vi "Populate Tree View.vi"(7 "Tree":refnum<vi>, 8 "error in (no error)":errorcluster, 11 "Element":refnum<class "Config Element.lvclass">) -> (0 "error out":errorcluster)   [LabVIEW 2020, in "CDM-Config.lvlib"]
doc: "Helper VI to populate a tree control with the specified config tree, starting with the specified [sub]tree root <b>Element</b>. This VI Defers Panel Updates on the owning VI of the <b>Tree</b> while updating the tree to increase performance."
uses:
  CDM-Config.lvlib
  Config Element/Config Element.lvclass
  Config Element/Config Element.lvclass/Config Element.ctl
  0270a6bc-9e24-4c23-b336-e1204a0f26d3.vi
  <vilib>/AdvancedString/1D String Array to Delimited String.vi
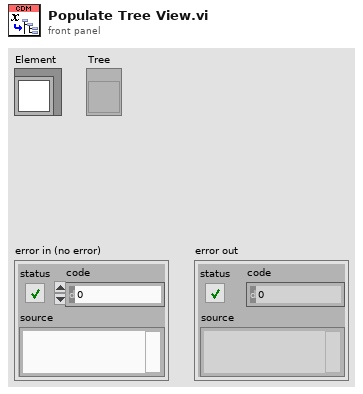
[diagram p1: front panel]
types:
  T1 = typedef "CDM-Config.lvlib/Meta Data.ctl" = cluster{"Name":string, "Value":string}
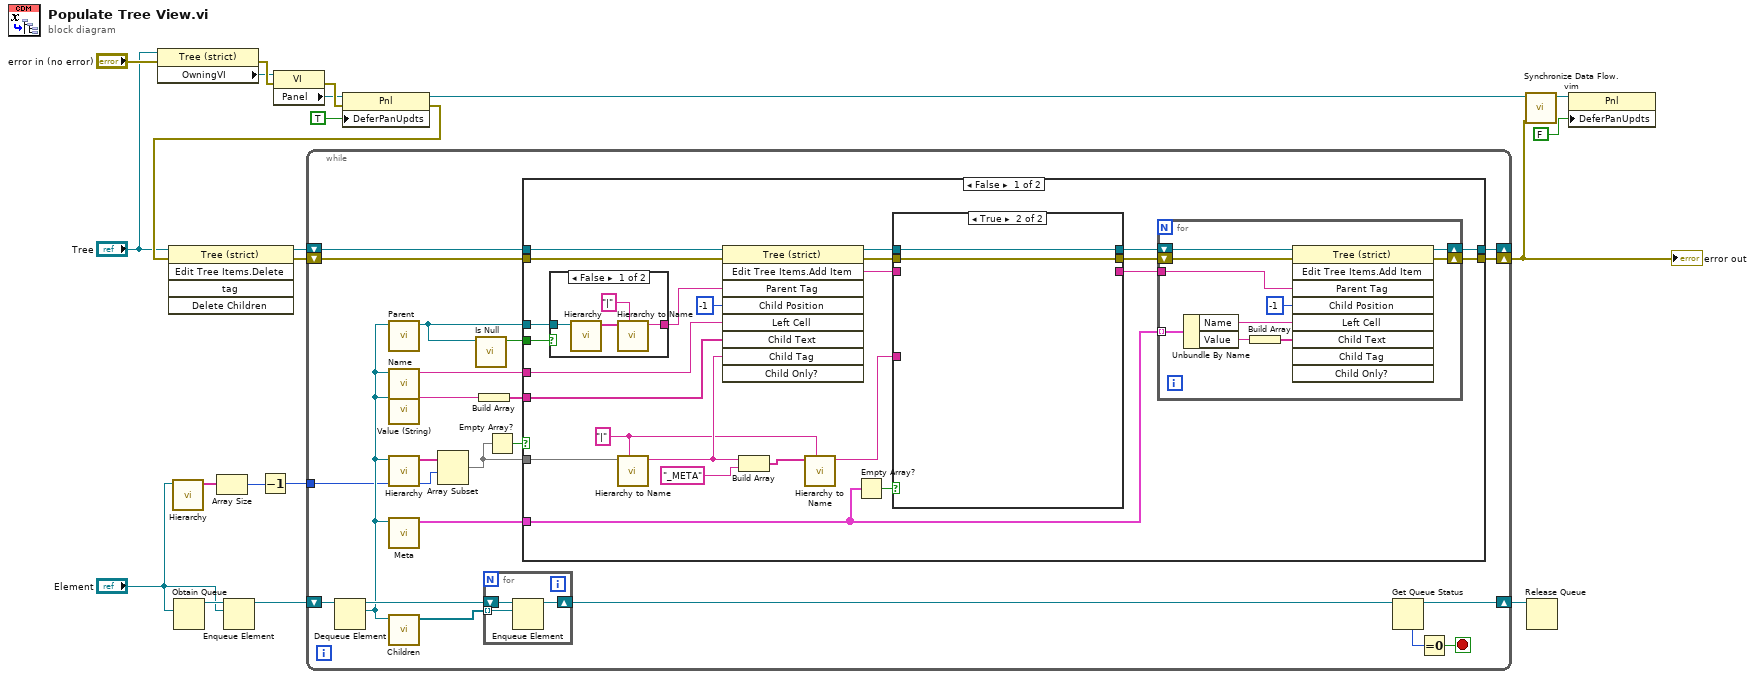
[diagram p0: block diagram]
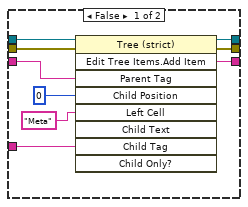
[diagram p3: hidden frame]
diagram:
  n1 = property class="Tree (strict)"(reference="Tree", error in="error in (no error)") -> (error out=w20:errorcluster, "OwningVI"=w12:refnum<vi>)  [unwired: 1 out]
  n2 = call "Hierarchy.vi"("Config Element in"="Element") -> ("Hierarchy"=w3:string[])  [unwired: 9 in, 1 out]
  n3 = Obtain Queue(element data type="Element") -> (queue out=w17:refnum<queue>)  [unwired: 4 in, 2 out]
  n4 = Array Size(array=w3) -> (size(s)=w2:i32)
  n5 = Enqueue Element(queue=w17, element="Element") -> (queue out=w16:refnum<queue>)  [unwired: 2 in, 2 out]
  n6 = Decrement(x=w2) -> (x-1=w1:i32)
  n7 = property class="VI"(reference=w12, error in=w20) -> (error out=w19:errorcluster, "Panel"=w11:refnum<vi>)  [unwired: 1 out]
  n8 = property class="Pnl"(reference=w11, error in=w19, "DeferPanUpdts"=TRUE ("Defer Panel Updates")) -> (reference out=w9:refnum<vi>, error out=w18:errorcluster)
  n9 = invoke class="Tree (strict)" method="Edit Tree Items.Delete"(reference="Tree", error in=w18) -> (reference out=w15:refnum<vi>, error out=w14:errorcluster)  [unwired: 3 in, 3 out]
  n10 = while {
    shift-right: [w42] -> w5
    shift-left: w16 -> [w43]
    shift-right: [w31] -> _
    shift-left: w15 -> [w36]
    shift-right: [w30] -> w7
    shift-left: w14 -> [w35]
    tunnel: w1 -> [w22]
    stop <- w39 stop-if-true
    n11 = Dequeue Element(queue=w43) -> (queue out=w41:refnum<queue>, element=w29:refnum<class "Config Element.lvclass">)  [unwired: 2 in, 2 out]
    n12 = call "Parent.vi"("Config Element in"=w29) -> ("Parent"=w33:refnum<class "Config Element.lvclass">)  [unwired: 9 in, 1 out]
    n13 = call "Name.vi"("Config Element in"=w29) -> ("Name"=w32:string)  [unwired: 9 in, 1 out]
    n14 = call "Value (String).vi"("Config Element in"=w29) -> ("String Value"=w28:string)  [unwired: 9 in, 1 out]
    n15 = call "Hierarchy.vi"("Config Element in"=w29) -> ("Hierarchy"=w24:string[])  [unwired: 9 in, 1 out]
    n16 = call "Meta.vi"("Config Element in"=w29) -> ("Meta Data"=w26:T1[])  [unwired: 9 in, 1 out]
    n17 = call "Children.vi"("Config Element in"=w29) -> ("Elements"=w37:refnum<class "Config Element.lvclass">[])  [unwired: 9 in, 1 out]
    n18 = Array Subset(array=w24, index=w22) -> (w23:string[])  [unwired: 1 in]
    n19 = call "Is Null.vi"("Config Element in"=w33) -> ("Null"=w34:bool)  [unwired: 10 in]
    n20 = Build Array(w28) -> (w27:string[])
    n21 = for {
      shift-right: [w96] -> w38
      shift-left: w41 -> [w97]
      tunnel: w37 -> [w95] mode=indexing
      n22 = Enqueue Element(queue=w97, element=w95) -> (queue out=w96:refnum<queue>)  [unwired: 2 in, 2 out]
    }
    n23 = Empty Array?(array=w23) -> (empty?=w25:bool)
    n24 = case shown="False" w25 {
      tunnel: w36 -> [w67 w94]
      tunnel: w35 -> [w66 w93]
      tunnel: w34 -> [w65 _]
      tunnel: w33 -> [w64 _]
      tunnel: w32 -> [w62 _]
      tunnel: [w61 w94] -> w31
      tunnel: [w60 w93] -> w30
      tunnel: w27 -> [w47 _]
      tunnel: w26 -> [w45 _]
      tunnel: w23 -> [w44 _]
      frame False {
        w52 = "|" ("Delimiter")
        n25 = case shown="False" w65 {
          tunnel: w64 -> [w69 _]
          tunnel: [w68 _] -> w63
          frame False {
            n26 = call "Hierarchy.vi"("Config Element in"=w69) -> ("Hierarchy"=w70:string[])  [unwired: 9 in, 1 out]
            n27 = call "Hierarchy to Name.vi"("Delimiter"="|", "Hierarchy"=w70) -> ("Full Name"=w68:string)  [unwired: 9 in]
          }
          frame True {
          }
        }
        n28 = call "Hierarchy to Name.vi"("Delimiter"=w52, "Hierarchy"=w44) -> ("Full Name"=w59:string)  [unwired: 9 in]
        n29 = invoke class="Tree (strict)" method="Edit Tree Items.Add Item"(reference=w67, error in=w66, "Parent Tag"=w63, "Child Position"=-1, "Left Cell"=w62, "Child Text"=w47, "Child Tag"=w59) -> (reference out=w56:refnum<vi>, error out=w55:errorcluster, "Edit Tree Items:Add Item"=w54:string)  [unwired: 2 in, 6 out]
        n30 = Build Array(w59, "_META" ("element")) -> (w53:string[])
        n31 = call "Hierarchy to Name.vi"("Delimiter"=w52, "Hierarchy"=w53) -> ("Full Name"=w51:string)  [unwired: 9 in]
        n32 = Empty Array?(array=w45) -> (empty?=w57:bool)
        n33 = case shown="True" w57 {
          tunnel: w56 -> [w80 w82]
          tunnel: w55 -> [w79 w81]
          tunnel: w54 -> [w78 _]
          tunnel: w51 -> [w73 _]
          tunnel: [w77 _] -> w50
          tunnel: [w76 w82] -> w49
          tunnel: [w75 w81] -> w48
          frame False {
            n34 = invoke class="Tree (strict)" method="Edit Tree Items.Add Item"(reference=w80, error in=w79, "Parent Tag"=w78, "Child Position"=0, "Left Cell"="Meta" ("Left Cell String"), "Child Tag"=w73) -> (reference out=w76:refnum<vi>, error out=w75:errorcluster, "Edit Tree Items:Add Item"=w77:string)  [unwired: 3 in, 6 out]
          }
          frame True {
          }
        }
        n35 = for {
          shift-right: [w87] -> w61
          shift-left: w49 -> [w91]
          shift-right: [w86] -> w60
          shift-left: w48 -> [w90]
          tunnel: w45 -> [w92] mode=indexing
          tunnel: w50 -> [w89]
          n36 = Unbundle By Name(w92) -> ("Name"=w88:string, "Value"=w85:string)
          n37 = Build Array(w85) -> (w84:string[])
          n38 = invoke class="Tree (strict)" method="Edit Tree Items.Add Item"(reference=w91, error in=w90, "Parent Tag"=w89, "Child Position"=-1, "Left Cell"=w88, "Child Text"=w84) -> (reference out=w87:refnum<vi>, error out=w86:errorcluster)  [unwired: 3 in, 7 out]
        }
      }
      frame True {
      }
    }
    n39 = Get Queue Status(queue=w38) -> (queue out=w42:refnum<queue>, # elements in queue=w40:i32)  [unwired: 2 in, 6 out]
    n40 = Equal To 0?(x=w40) -> (x = 0?=w39:bool)
  }
  "error out" <- w7
  n41 = call "Synchronize Data Flow.vim"("input 4"=w7, "input 1"=w9) -> ("output 1"=w8:refnum<vi>)  [unwired: 2 in, 3 out]
  n42 = Release Queue(queue=w5) -> ()  [unwired: 2 in, 3 out]
  n43 = property class="Pnl"(reference=w8, "DeferPanUpdts"=FALSE ("Defer Panel Updates")) -> ()  [unwired: 1 in, 2 out]
